vi "UMLEditor_OnHotSpot.vi"(7 "ZoomLevel":dbl, 8 "error in (no error)":errorcluster, 9 "ObjectHotspots":T2[](array[typedef]) {"HotSpot"."y" format="%.2f"; "HotSpot"."x" format="%.2f"}, 10 "Mouse Position":cluster{"X":i32, "Y":i32}) -> (0 "error out":errorcluster, 1 "Function":T1, 2 "HotSpotCursor":bool, 3 "Node":refnum<class "AbstractNode.lvclass">)   [LabVIEW 2020]
uses:
  <resource>/Framework/Providers/Open_GDS/UML/UMLEditor/UMLEditor_HotSpotData.ctl
  <resource>/Framework/Providers/Open_GDS/UML/AbstractNode_class/AbstractNode.lvclass
  <resource>/Framework/Providers/Open_GDS/UML/General/Point/Point Point2D.ctl
  <resource>/Framework/Providers/Open_GDS/UML/UMLEditor/UMLEditor_HotSpotType.ctl
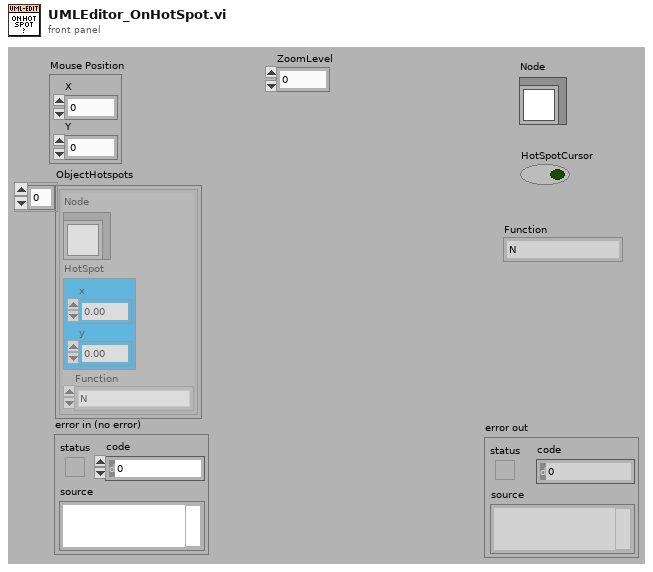
[diagram p1: front panel]
types:
  T1 = typedef "UMLEditor_HotSpotType.ctl" = enum16{"N", "NE", "E", "SE", "S", "SW", "W", "NW", "Expand", "Collaps"}
  T2 = typedef "UMLEditor_HotSpotData.ctl" = cluster{"Node":refnum<class "AbstractNode.lvclass">, "HotSpot":T3, "Function":T1}
  T3 = typedef "Point Point2D.ctl" = cluster{"x":dbl, "y":dbl}
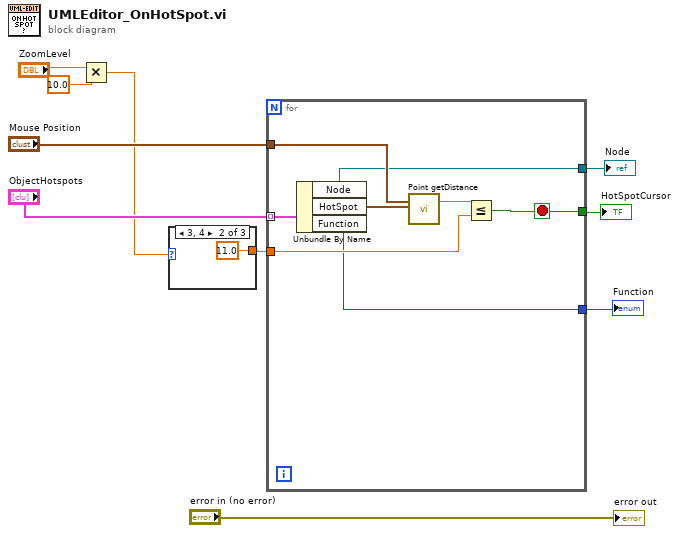
[diagram p0: block diagram]
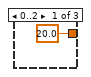
[diagram p2: hidden frame]
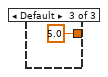
[diagram p3: hidden frame]
diagram:
  n1 = Multiply(x="ZoomLevel", y=10.0) -> (x*y=w1:dbl)
  n2 = case shown="3, 4" w1 {
    tunnel: [20.0 ("y") 11.0 ("y") 5.0 ("y")] -> w10
    frame 0..2 {
    }
    frame 3, 4 {
    }
    frame Default {
    }
  }
  n3 = for {
    tunnel: w10 -> [w18]
    tunnel: [w16] -> w7
    tunnel: [w17] -> w8
    tunnel: "ObjectHotspots" -> [w21] mode=indexing
    tunnel: "Mouse Position" -> [w15]
    tunnel: [w14] -> w4
    stop <- w17 stop-if-true
    n4 = Unbundle By Name(w21) -> ("Node"=w14:refnum<class "AbstractNode.lvclass">, "HotSpot"=w20:T3, "Function"=w16:T1)
    n5 = call <resource>:"Point getDistance.vi"("point1"=w15, "point2"=w20) -> ("distance"=w19:dbl)  [unwired: 16 in, 1 out]
    n6 = Less Or Equal?(x=w19, y=w18) -> (x <= y?=w17:bool)
  }
  "Function" <- w7
  "HotSpotCursor" <- w8
  "Node" <- w4
  "error out" <- "error in (no error)"
